vi "RT-Terminate.vi"(1 "Motor Controller":T2, 2 "Data input":T1) -> ()   [LabVIEW 2020]
uses:
  <vilib>/FPGAPlugInAG/Dynamic/niLvFpga_Close_Dynamic.vi
  <vilib>/rvi/interface/nirviCloseFPGA/nirviCloseFPGA.xnode
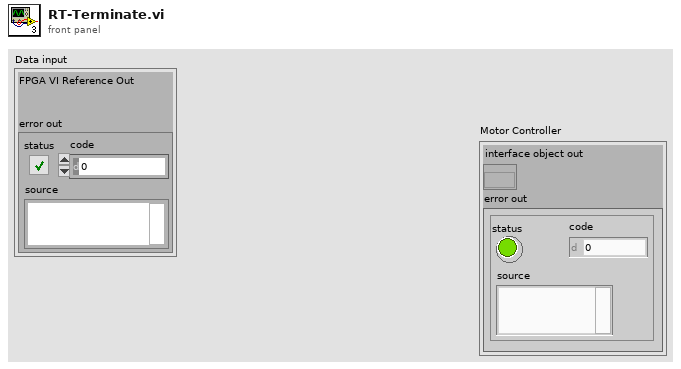
[diagram p1: front panel]
types:
  T1 = cluster{"FPGA VI Reference Out":refnum<k20>, "error out":errorcluster}
  T2 = cluster{"interface object out":refnum<k20>, "error out":errorcluster}
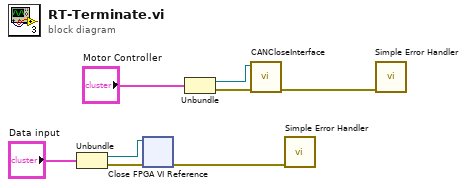
[diagram p0: block diagram]
diagram:
  n1 = Unbundle "Unbundle"("Data input") -> ("FPGA VI Reference Out"=w4:refnum<k20>, "error out"=w3:errorcluster)
  n2 = xnode "Close FPGA VI Reference"("FPGA VI Reference In"=w4, "error in"=w3) -> ("error out"=w2:errorcluster)
  n3 = Unbundle "Unbundle"("Motor Controller") -> ("interface object out"=w8:refnum<k20>, "error out"=w6:errorcluster)
  n4 = call <vilib>:"CANCloseInterface.vi"("error in (no error)"=w6, "interface object in"=w8) -> ("error out"=w5:errorcluster)  [unwired: 9 in]
  n5 = call <vilib>:"Simple Error Handler.vi"("error in (no error)"=w2) -> ()  [unwired: 4 in, 5 out]
  n6 = call <vilib>:"Simple Error Handler.vi"("error in (no error)"=w5) -> ()  [unwired: 4 in, 5 out]
